vi "Convert DBL to string-decimal precision.vi"(9 "Format (%f)":string="%f", 11 "DBL Value":dbl) -> (3 "Converted to String":string)   [LabVIEW 2017]
uses:
  <userlib>/_OpenG.lib/string/string.llb/Trim Whitespace (String Array)__ogtk.vi
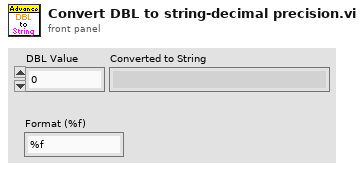
[diagram p1: front panel]
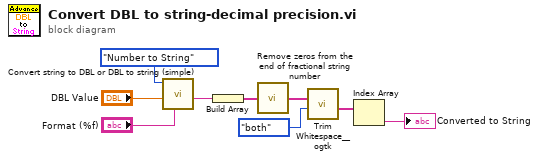
[diagram p0: block diagram]
diagram:
  n1 = call "Convert string to DBL or DBL to string (simple).vi"("Format"="Format (%f)", "Number in (DBL)"="DBL Value", "Mode"=enum16{"String to Number", "Number to String"}."Number to String") -> ("String out"=w4:string)  [unwired: 7 in, 1 out]
  n2 = Build Array(w4) -> (w5:string[])
  n3 = call "Remove zeros from the end of fractional string number.vi"("Strings Array"=w5) -> ("Filtered Strings Array"=w3:string[])
  n4 = call-poly <userlib>:"Trim Whitespace__ogtk.vi"("remove (leading and trailing)"=enum16{"leading", "trailing", "both"}."both", "String in"=w3) -> ("String out"=w6:string[])  [unwired: 5 in]
  n5 = Index Array(array=w6) -> (element=→"Converted to String":string)  [unwired: 1 in]
